vi "Day 1 Task 2.vi"() -> ()   [LabVIEW 2018]
panel:
  out "Log of window":string[](array[string])
  out "sums":i32[](array[numeric])
  out "sum":i16
  out "array w/ subset deleted":bool[](array[boolean])
  out "Log":string[](array[string])
  out "Array":bool[](array[boolean])
  out "Sea floor depths":i32[](array[numeric])
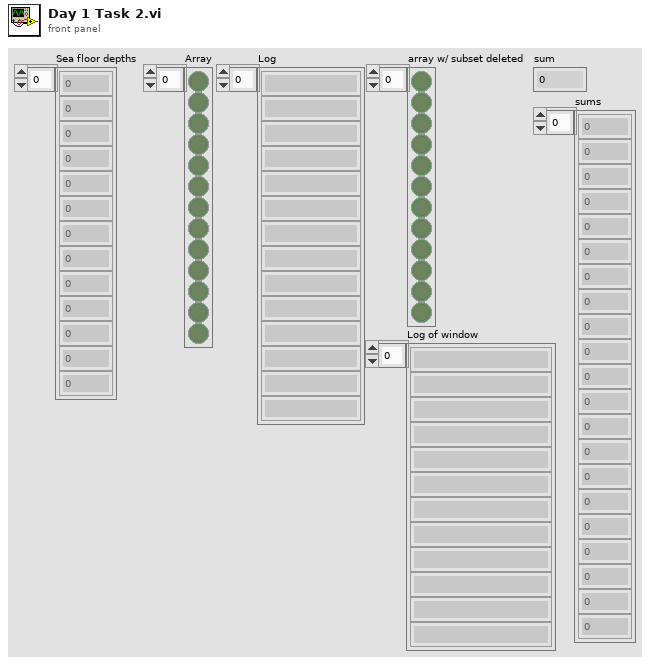
[diagram p1: front panel]
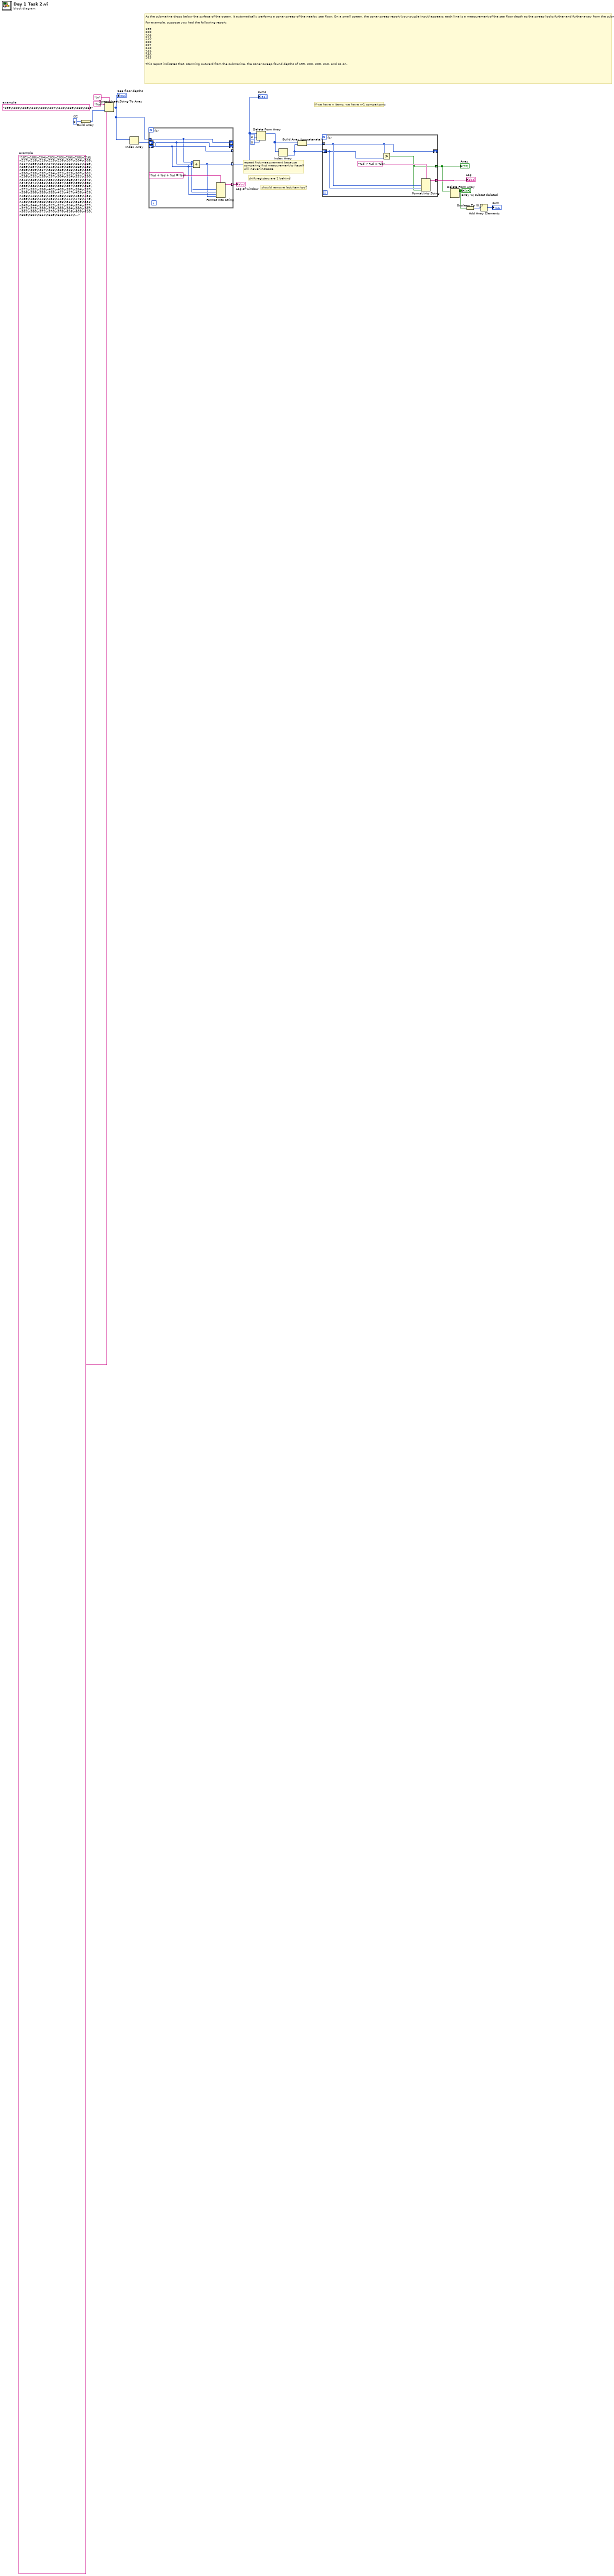
[diagram p0: block diagram]
diagram:
  w1 = "182\n188\n204\n203\n205\n206\n208\n216\n217\n218\n219\n225\n226\n207\n204\n205\n217\n255\n254\n270\n261\n262\n264\n265\n255\n257\n249\n248\n249\n250\n265\n286\n308\n309\n317\n326\n328\n316\n318\n333\n330\n293\n292\n294\n321\n313\n307\n301\n296\n291\n295\n297\n304\n314\n331\n330\n342\n325\n324\n354\n360\n368\n371\n372\n373\n374\n381\n384\n387\n389\n390\n392\n393\n382\n361\n350\n356\n357\n359\n363\n371\n391\n398\n402\n403\n397\n394\n397\n396\n398\n399\n393\n411\n417\n428\n429\n456\n446\n451\n459\n456\n460\n458\n451\n455\n452\n446\n451\n448\n444\n476\n478\n480\n503\n502\n504\n496\n511\n518\n531\n543\n544\n516\n512\n511\n514\n524\n522\n523\n535\n558\n576\n589\n584\n580\n582\n581\n580\n571\n570\n578\n616\n609\n610\n603\n604\n614\n615\n616\n614\n..."  # example
  w16 = 0  # i32
  (unwired) "199\n200\n208\n210\n200\n207\n240\n269\n260\n263"  # example
  # "shift registers are 1 behind"
  # "should remove last item too?"
  # "If we have n items, we have n-1 comparisons"
  # "repeat first measurement because\ncomparing first measurement to iteself\nwill never increase"
  # "As the submarine drops below the surface of the ocean, it automatically performs a sonar sweep of the nearby sea floor. On a small screen, the sonar sweep report (your puzzle input) appears: each line is a measurement of the sea floor depth as the sweep looks further and further away from the submarine.\n\nFor example, suppose you had the following report:\n\n199\n200\n208\n210\n200\n207\n240\n269\n260\n263\n\nThis report indicates that, scanning outward from the submarine, the sonar sweep found depths of 199, 200, 208, 210, and so on."
  n1 = Build Array(w16) -> (w17:i32[])
  n2 = Spreadsheet String To Array(delimiter (Tab)="\n", format string="%d", spreadsheet string=w1, array type (2D Dbl)=w17) -> (array=w7:i32[])
  "Sea floor depths" <- w7
  n3 = Index Array(array=w7) -> (element=w8:i32)  [unwired: 1 in]
  n4 = for {
    tunnel: w7 -> [w22] mode=indexing
    shift-right: [w22] -> _
    shift-left: w8 -> [w23]
    shift-right: [w23] -> _
    shift-left: w8 -> [w24]
    tunnel: [w24] -> _ mode=indexing
    tunnel: [w20] -> w5 mode=indexing
    tunnel: [w21] -> w6 mode=indexing
    n5 = Compound Arithmetic op=ADD(w22, w23, w24) -> (w20:i32)
    n6 = Format Into String(format string="%d + %d + %d = %d", w22, w23, w24, w20) -> (resulting string=w21:string)  [unwired: 2 in, 1 out]
  }
  "sums" <- w5
  "Log of window" <- w6
  n7 = Delete From Array(array=w5, length=2, index=0) -> (array with subset deleted=w2:i32[])  [unwired: 1 out]
  n8 = Index Array(array=w2) -> (element=w14:i32)  [unwired: 1 in]
  n9 = Build Array (concatenate)(w2, w14) -> (w15:i32[])
  n10 = for {
    tunnel: w15 -> [w29] mode=indexing
    shift-right: [w29] -> _
    shift-left: w14 -> [w28]
    tunnel: [w27] -> w12 mode=indexing
    tunnel: [w26] -> w13 mode=indexing
    n11 = Greater?(x=w29, y=w28) -> (0:w27:bool)
    n12 = Format Into String(format string="%d > %d = %b", w29, w28, w27) -> (resulting string=w26:string)  [unwired: 2 in, 1 out]
  }
  "Array" <- w12
  "Log" <- w13
  n13 = Delete From Array(array=w12) -> (array with subset deleted=w11:bool[])  [unwired: 2 in, 1 out]
  "array w/ subset deleted" <- w11
  n14 = Boolean To (0,1)(Boolean=w11) -> (0, 1=w10:i16[])
  n15 = Add Array Elements(numeric array=w10) -> (sum=→"sum":i16)
